vi "Schedule Ore Robot.vi"(6 "max geodes in":u8=24, 7 "max time in":u8=24, 8 "costs in":T1, 9 "data value reference":refnum<data-value>, 10 "stack in":refnum<queue>, 11 "mine in":refnum<class "Mine.lvclass">) -> (0 "costs out":T1, 1 "data value reference":refnum<data-value>, 2 "stack out":refnum<queue>, 3 "mine out":refnum<class "Mine.lvclass">, 4 "max geodes out":u8, 5 "max time out":u8)   [LabVIEW 2021, in "d19.lvlib" / "Mine.lvclass"]
uses:
  Mine.lvclass
  Mine.lvclass/Mine.ctl
  <vilib>/Utility/miscctls.llb/LVMapReplaceAction.ctl
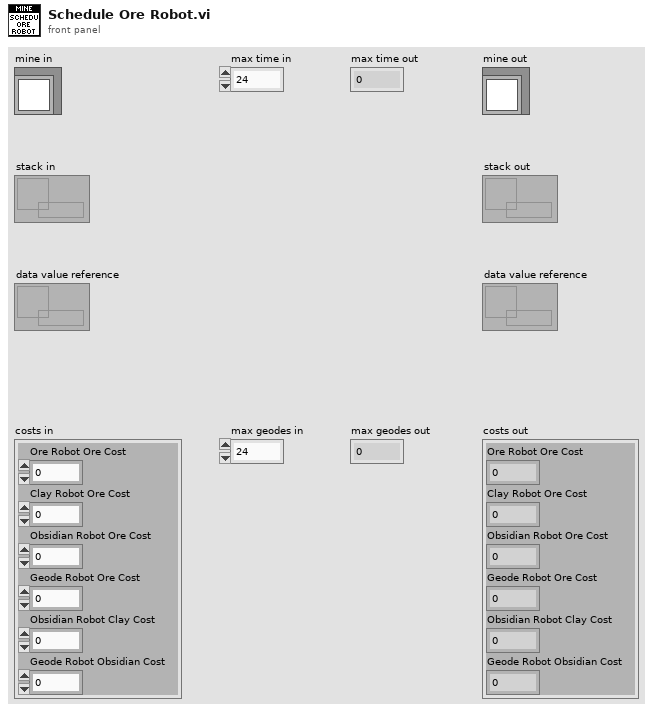
[diagram p1: front panel]
types:
  T1 = cluster{"Ore Robot Ore Cost":u8, "Clay Robot Ore Cost":u8, "Obsidian Robot Ore Cost":u8, "Geode Robot Ore Cost":u8, "Obsidian Robot Clay Cost":u8, "Geode Robot Obsidian Cost":u8}
  T2 = typedef "LVMapReplaceAction.ctl" = enum32{"Modify Entry only if found", "Add or Modify Entry", "Delete Entry"}
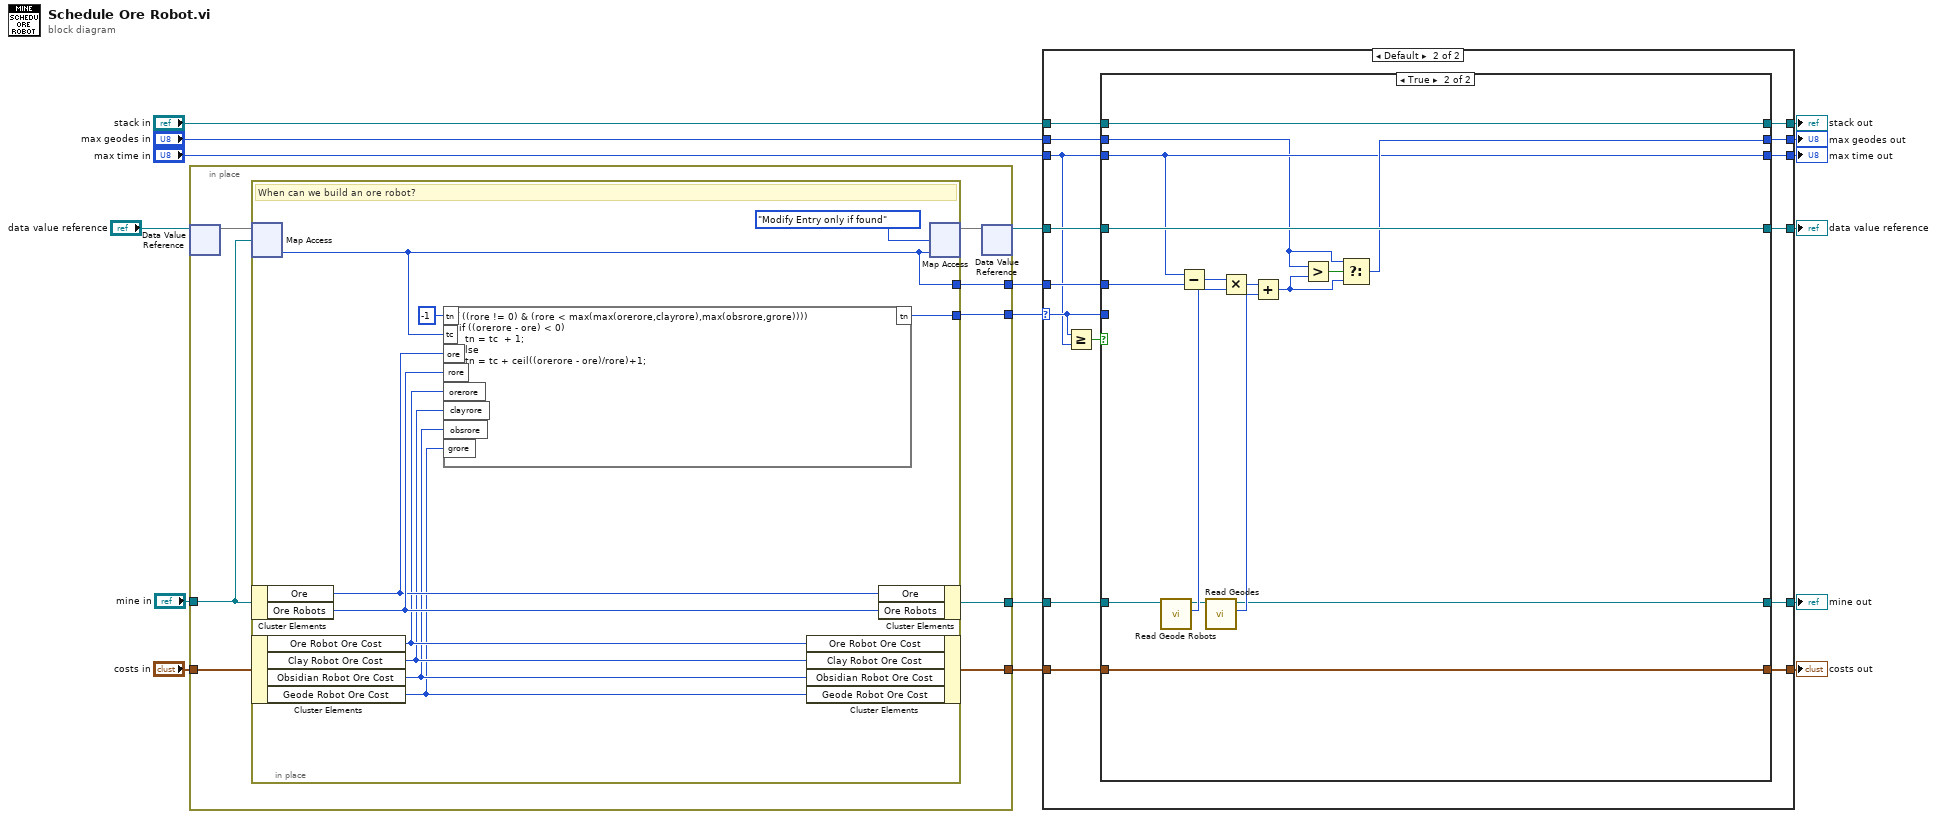
[diagram p0: block diagram]
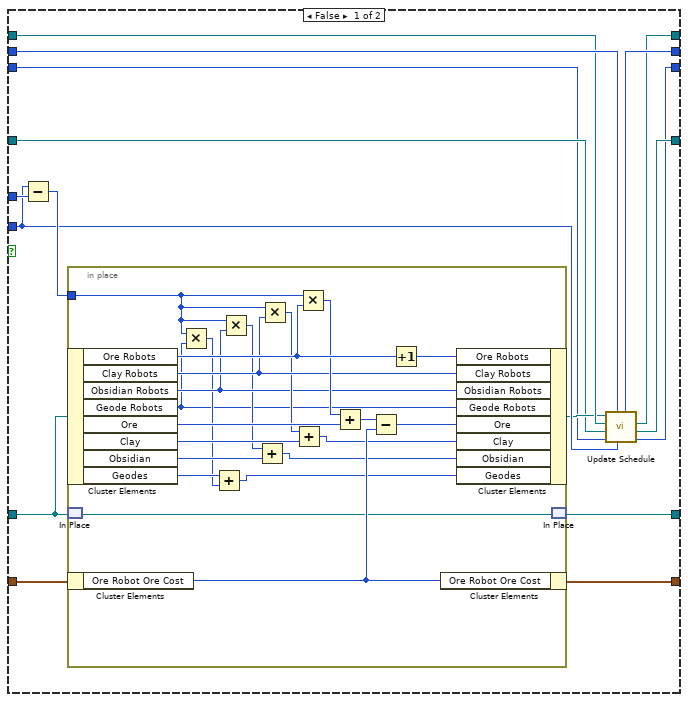
[diagram p3: hidden frame]
diagram:
  n1 = in-place {
    in-place-border: [w25] -> w17
    in-place-border: [w24] -> w7
    in-place-border: "mine in" -> [w23]
    in-place-border: "costs in" -> [w22]
    in-place-border: [w21] -> w4
    in-place-border: [w20] -> w3
    n2 = in-place-dvr #1("data value reference") -> (w19:map{refnum<class "Mine.lvclass">, u8})  [unwired: 1 out]
    n3 = in-place {
      in-place-border: [w34] -> w25
      in-place-border: [w32] -> w24
      # "When can we build an ore robot?"
      n4 = in-place-map #2(w19, w23) -> (w32:u8)  [unwired: 1 in, 1 out]
      n5 = in-place-cluster #3(w23) -> ("Ore"=w30:u8, "Ore Robots"=w31:u8)
      n6 = in-place-cluster #4(w22) -> ("Ore Robot Ore Cost"=w29:u8, "Clay Robot Ore Cost"=w28:u8, "Obsidian Robot Ore Cost"=w27:u8, "Geode Robot Ore Cost"=w26:u8)
      n7 = formula code="if ((rore != 0) & (rore < max(max(orerore,clayrore),max(obsrore,grore))))\n  if ((orerore - ore) < 0)\n    tn = tc  + 1;\n  else\n    tn = tc + ceil((orerore - ore)/rore)+1;"("tc"=w32, "orerore"=w29, "clayrore"=w28, "ore"=w30, "rore"=w31, "tn"=i8 -1, "obsrore"=w27, "grore"=w26) -> ("tn"=w34:i8)
      n8 = in-place-cluster #4("Ore Robot Ore Cost"=w29, "Clay Robot Ore Cost"=w28, "Obsidian Robot Ore Cost"=w27, "Geode Robot Ore Cost"=w26) -> (w20:T1)
      n9 = in-place-cluster #3("Ore"=w30, "Ore Robots"=w31) -> (w21:refnum<class "Mine.lvclass">)
      n10 = in-place-map #2(w32, LVMapReplaceAction."Modify Entry only if found" ("action")) -> (w18:map{refnum<class "Mine.lvclass">, u8})  [unwired: 2 out]
    }
    n11 = in-place-dvr #1(w18) -> (w1:refnum<data-value>)  [unwired: 1 out]
  }
  n12 = case shown="Default" w17 {
    selector: w17 -> [_ w44]
    tunnel: "stack in" -> [w41 w56]
    tunnel: [w41 w55] -> w15
    tunnel: [w38 w54] -> w14
    tunnel: [w36 w53] -> w13
    tunnel: [w37 w52] -> w12
    tunnel: "max time in" -> [w39 w43]
    tunnel: "max geodes in" -> [w40 w51]
    tunnel: [w40 w50] -> w9
    tunnel: [w39 w49] -> w8
    tunnel: w7 -> [_ w48]
    tunnel: w4 -> [w37 w47]
    tunnel: w3 -> [w36 w46]
    tunnel: w1 -> [w38 w45]
    frame -1 {
    }
    frame Default {
      n13 = Greater Or Equal?(x=w44, y=w43) -> (x >= y?=w42:bool)
      n14 = case shown="True" w42 {
        tunnel: w45 -> [w61 w109]
        tunnel: [w59 w109] -> w54
        tunnel: w56 -> [w63 w108]
        tunnel: [w58 w108] -> w55
        tunnel: w46 -> [w72 w107]
        tunnel: w47 -> [w70 w97]
        tunnel: [w71 w107] -> w53
        tunnel: [w69 w95] -> w52
        tunnel: w43 -> [w60 w103]
        tunnel: w51 -> [w68 w94]
        tunnel: [w67 w105] -> w50
        tunnel: [w57 w103] -> w49
        tunnel: w48 -> [w66 w102]
        tunnel: w44 -> [w64 _]
        frame False {
          n15 = Subtract(x=w64, y=w66) -> (x-y=w65:u8)
          n16 = in-place {
            in-place-border: w65 -> [w77]
            n17 = in-place-cluster #5(w70) -> ("Ore Robots"=w87:u8, "Clay Robots"=w83:u8, "Obsidian Robots"=w81:u8, "Geode Robots"=w75:u8, "Ore"=w93:u8, "Clay"=w90:u8, "Obsidian"=w80:u8, "Geodes"=w89:u8)
            n18 = in-place-match #6(w70) -> (w88:refnum<class "Mine.lvclass">)
            n19 = in-place-cluster #7(w72) -> ("Ore Robot Ore Cost"=w92:u8)
            n20 = Multiply(x=w77, y=w75) -> (x*y=w76:u8)
            n21 = Add(x=w89, y=w76) -> (x+y=w74:u8)
            n22 = Multiply(x=w77, y=w81) -> (x*y=w78:u8)
            n23 = Add(x=w78, y=w80) -> (x+y=w79:u8)
            n24 = Multiply(x=w77, y=w83) -> (x*y=w82:u8)
            n25 = Add(x=w82, y=w90) -> (x+y=w85:u8)
            n26 = Multiply(x=w77, y=w87) -> (x*y=w84:u8)
            n27 = Add(x=w84, y=w93) -> (x+y=w86:u8)
            n28 = Subtract(x=w86, y=w92) -> (x-y=w91:u8)
            n29 = Increment(x=w87) -> (x+1=w73:u8)
            n30 = in-place-cluster #7("Ore Robot Ore Cost"=w92) -> (w71:T1)
            n31 = in-place-cluster #5("Ore Robots"=w73, "Clay Robots"=w83, "Obsidian Robots"=w81, "Geode Robots"=w75, "Ore"=w91, "Clay"=w85, "Obsidian"=w79, "Geodes"=w74) -> (w62:refnum<class "Mine.lvclass">)
            n32 = in-place-match #6(w88) -> (w69:refnum<class "Mine.lvclass">)
          }
          n33 = call "Update Schedule.vi"("new time"=w64, "max geodes in"=w68, "max time in"=w60, "map in"=w61, "stack in"=w63, "Mine in"=w62) -> ("max time out"=w57:u8, "map out"=w59:refnum<data-value>, "stack out"=w58:refnum<queue>, "max geodes out"=w67:u8)  [unwired: 1 in, 1 out]
        }
        frame True {
          n34 = call "Read Geode Robots.vi"("Mine in"=w97) -> ("Geode Robots"=w101:u8, "Mine out"=w96:refnum<class "Mine.lvclass">)  [unwired: 9 in]
          n35 = Subtract(x=w103, y=w102) -> (x-y=w100:u8)
          n36 = call "Read Geodes.vi"("Mine in"=w96) -> ("Geodes"=w104:u8, "Mine out"=w95:refnum<class "Mine.lvclass">)  [unwired: 9 in]
          n37 = Multiply(x=w100, y=w101) -> (x*y=w98:u8)
          n38 = Add(x=w98, y=w104) -> (x+y=w99:u8)
          n39 = Greater?(x=w94, y=w99) -> (0:w106:bool)
          n40 = Select(t=w94, s=w106, f=w99) -> (s? t:f=w105:u8)
        }
      }
    }
  }
  "stack out" <- w15
  "data value reference" <- w14
  "costs out" <- w13
  "mine out" <- w12
  "max geodes out" <- w9
  "max time out" <- w8
